vi "ConvertDLPVAGainStages.vi"(1 "Gain_2 i":bool, 2 "Gain_1 i":bool) -> (0 "Array":bool[](array[boolean]))   [LabVIEW 2010]
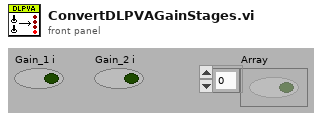
[diagram p1: front panel]
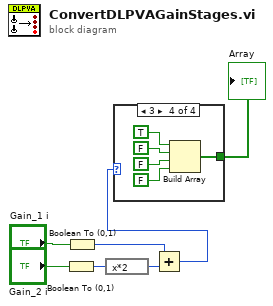
[diagram p0: block diagram]
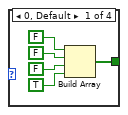
[diagram p2: hidden frame]
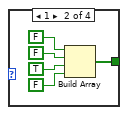
[diagram p3: hidden frame]
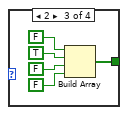
[diagram p4: hidden frame]
diagram:
  n1 = Boolean To (0,1)(Boolean="Gain_2 i") -> (0, 1=w4:i16)
  n2 = Boolean To (0,1)(Boolean="Gain_1 i") -> (0, 1=w6:i16)
  n3 = expression code="x*2"(w4) -> (w5:i16)
  n4 = Add(x=w6, y=w5) -> (x+y=w1:i16)
  n5 = case shown="3" w1 {
    tunnel: [w8 w13 w18 w23] -> w7
    frame 0, Default {
      n6 = Build Array(FALSE ("new element/subarray"), FALSE ("new element/subarray"), FALSE ("new element/subarray"), TRUE ("new element/subarray")) -> (w8:bool[])
    }
    frame 1 {
      n7 = Build Array(FALSE ("new element/subarray"), FALSE ("new element/subarray"), TRUE ("new element/subarray"), FALSE ("new element/subarray")) -> (w13:bool[])
    }
    frame 2 {
      n8 = Build Array(FALSE ("new element/subarray"), TRUE ("new element/subarray"), FALSE ("new element/subarray"), FALSE ("new element/subarray")) -> (w18:bool[])
    }
    frame 3 {
      n9 = Build Array(TRUE ("new element/subarray"), FALSE ("new element/subarray"), FALSE ("new element/subarray"), FALSE ("new element/subarray")) -> (w23:bool[])
    }
  }
  "Array" <- w7
